vi "Measure Frequency.vi"(8 "error in":errorcluster, 11 "Waveform":waveform(dbl)={"t0"=timestamp(0 s since 1904-01-01), "dt"=0.0, "Y"=[]}) -> (0 "error out":errorcluster, 1 "Vpeak":dbl, 2 "frequency":dbl, 3 "exported spectrum (dB)":T1)   [LabVIEW 2018]
doc: "Measure frequency of input signal."
uses:
  <vilib>/measure/matone.llb/Extract Single Tone Information 1 Chan.vi
  <vilib>/measure/NI_MAPro.lvlib
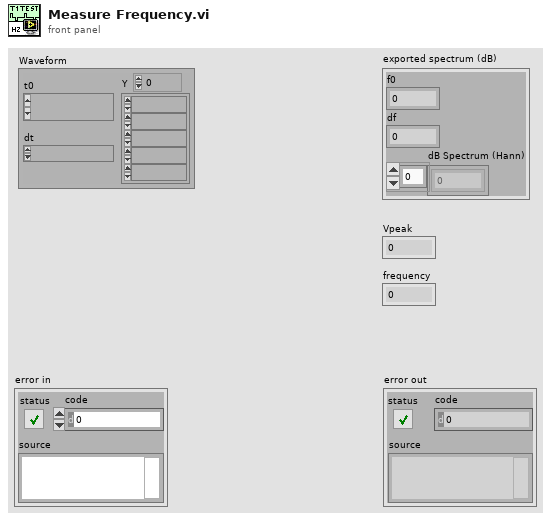
[diagram p1: front panel]
types:
  T1 = cluster{"f0":dbl, "df":dbl, "dB Spectrum (Hann)":dbl[]}
  T2 = enum32{"none", "input signal", "detected signal", "residual signal"}
  T3 = cluster{"approx freq. (optional)":dbl, "search (+/- % of Fsampl.)":dbl}
  T4 = cluster{"exported time signal":waveform(dbl), "exported spectrum (dB)":cluster{"f0":dbl, "df":dbl, "dB Spectrum (Hann)":dbl[]}}
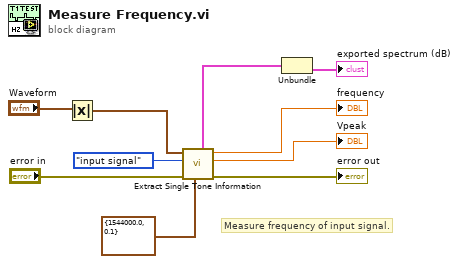
[diagram p0: block diagram]
diagram:
  # "Measure frequency of input signal."
  n1 = Absolute Value(x="Waveform") -> (abs(x)=w9:waveform(dbl))
  n2 = call-poly <vilib>:"Extract Single Tone Information.vi"("advanced search"=T3 {"approx freq. (optional)"=1544000.0, "search (+/- % of Fsampl.)"=0.1}, "error in (no error)"="error in", "export mode"=T2."input signal", "time signal in"=w9) -> ("error out"=→"error out":errorcluster, "detected amplitude"=→"Vpeak":dbl, "detected frequency"=→"frequency":dbl, "exported signals"=w7:T4)  [unwired: 2 in, 2 out]
  n3 = Unbundle(w7) -> ("exported spectrum (dB)"=→"exported spectrum (dB)":T1)  [unwired: 1 out]
